vi "Acquisition Message Loop.vi"(8 "error in (no error)":errorcluster, 9 "Data Queue":refnum<queue>, 10 "Data Notifier":refnum<notifier>, 11 "Message Queues":T1) -> (0 "error out":errorcluster)   [LabVIEW 2017, in "Acquisition.lvlib"]
doc: "Message loop for handling messages pertaining to the acquisition of data from the hardware."
uses:
  Acquisition.lvlib
  support/Message Queue/All Message Queues.ctl
  support/Message Queue/Message Cluster.ctl
  Hardware Configuration.ctl
  <vilib>/DAQmx/read.llb/DAQmx Read (Analog 1D Wfm NChan NSamp).vi
  support/Message Queue/Enqueue Message (Single).vi
  <vilib>/DAQmx/miscellaneous.llb/DAQmx Fill In Error Info.vi
  <vilib>/Utility/error.llb/Error Cluster From Error Code.vi
  <vilib>/ErrorRing/Error Ring.xnode
  support/Message Queue/Message Queue.lvlib
  <resource>/objmgr/daqmx.rc
panel:
  out "# waiting":i32
  out "# elements in queue":i32
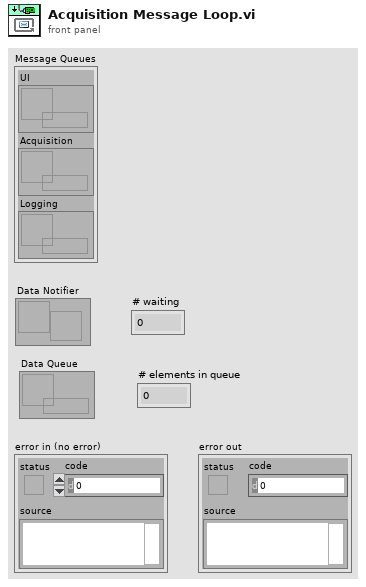
[diagram p1: front panel]
types:
  T1 = typedef "Message Queue.lvlib/All Message Queues.ctl" = cluster{"UI":refnum<queue>, "Acquisition":refnum<queue>, "Logging":refnum<queue>}
  T2 = typedef "Acquisition.lvlib/Hardware Configuration.ctl" = cluster{"DAQmx Input":tag, "Max Input":dbl, "Min Input":dbl, "Sample Rate":dbl, "DAQmx Task":refnum<k21>}
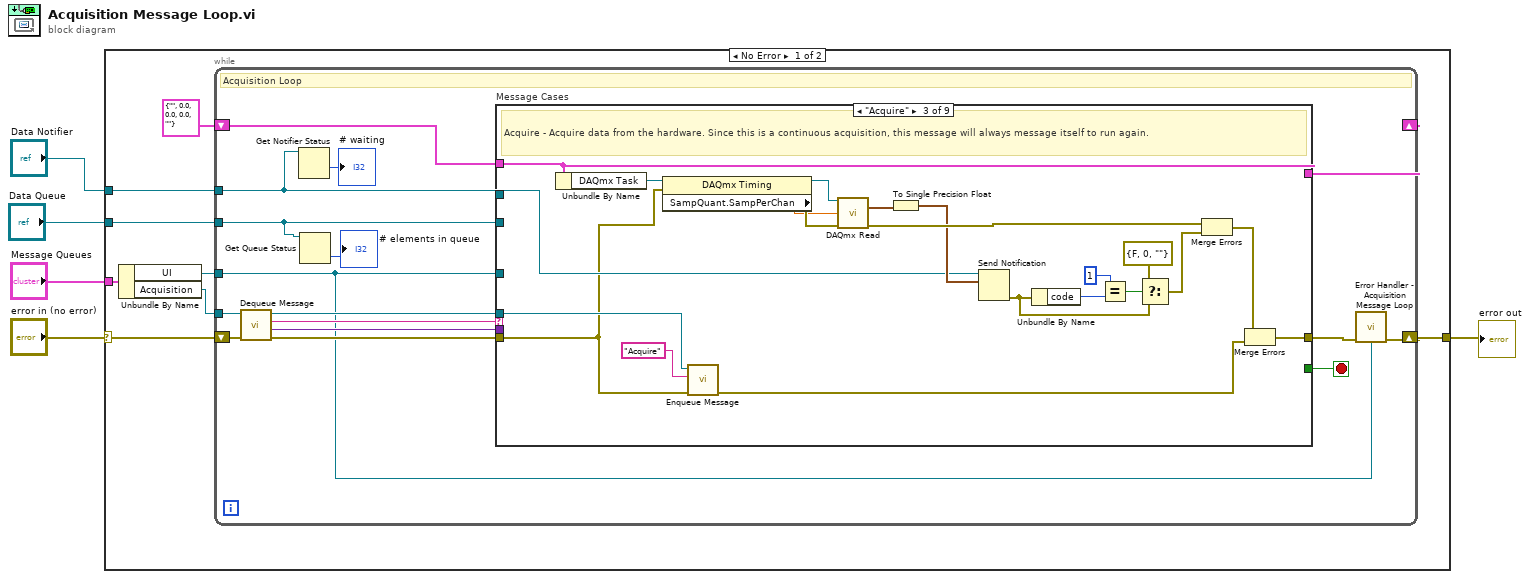
[diagram p0: block diagram]
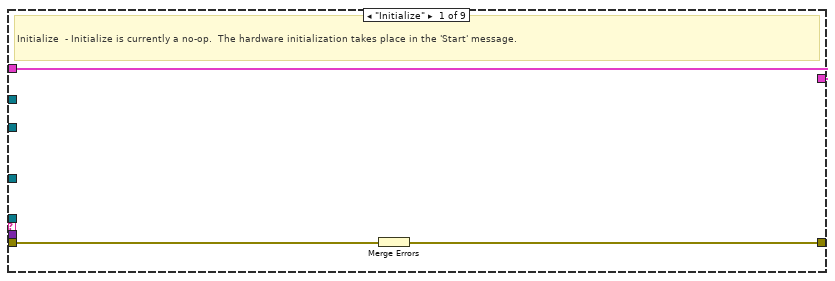
[diagram p2: hidden frame]
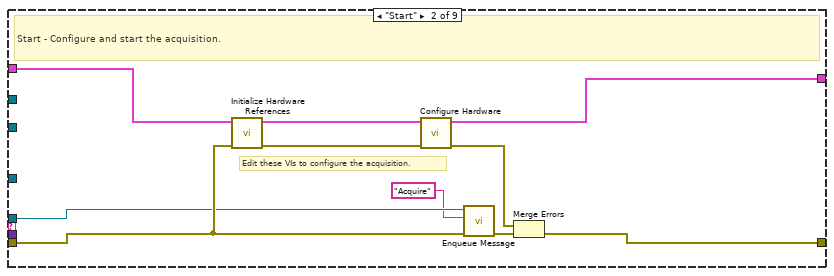
[diagram p3: hidden frame]
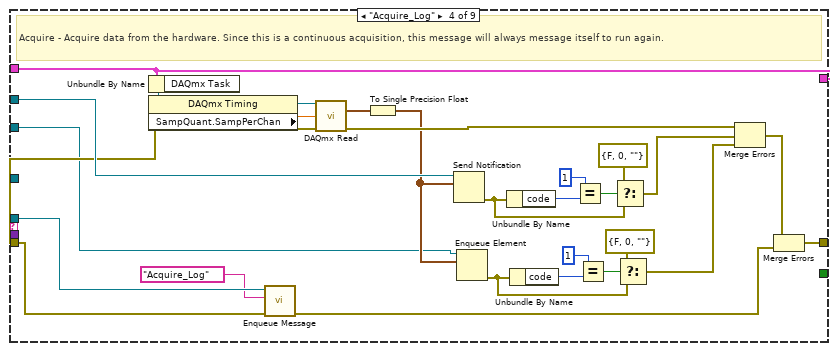
[diagram p4: hidden frame]
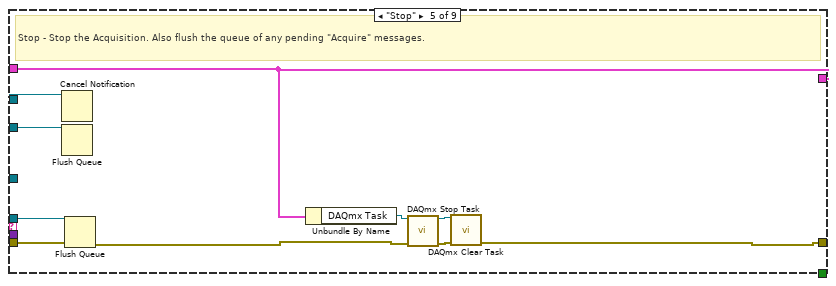
[diagram p5: hidden frame]
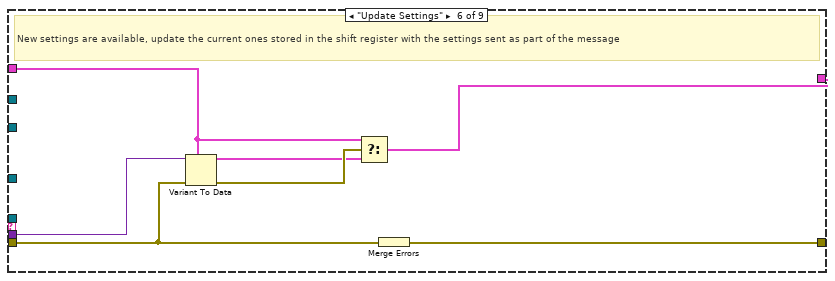
[diagram p6: hidden frame]
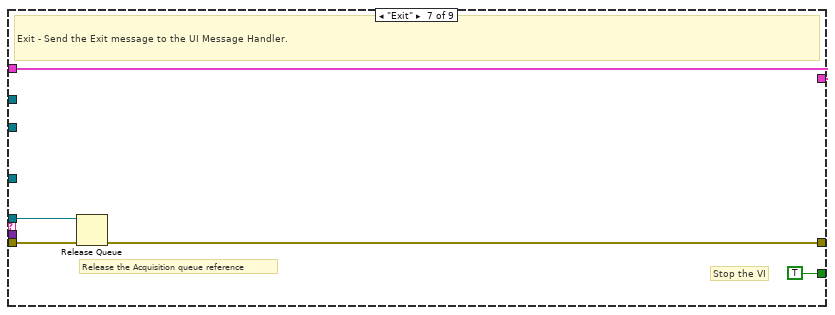
[diagram p7: hidden frame]
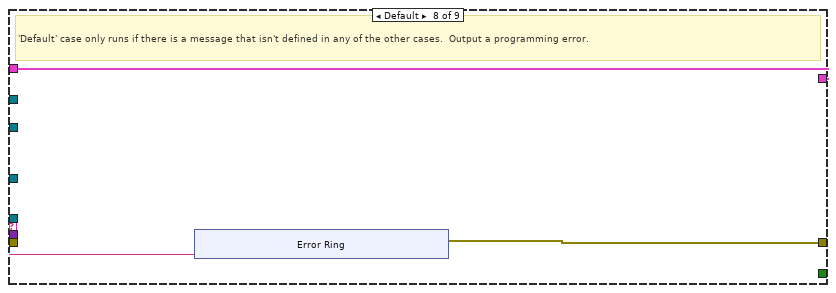
[diagram p8: hidden frame]
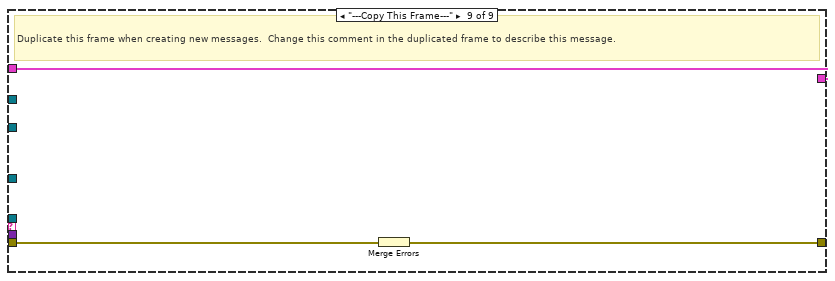
[diagram p9: hidden frame]
diagram:
  n1 = case shown="No Error" "error in (no error)" {
    selector: "error in (no error)" -> [w9 w127]
    tunnel: "Message Queues" -> [w13 _]
    tunnel: [w11 w127] -> w4
    tunnel: "Data Notifier" -> [w7 _]
    tunnel: "Data Queue" -> [w6 _]
    frame No Error {
      n2 = Unbundle By Name(w13) -> ("UI"=w8:refnum<queue>, "Acquisition"=w12:refnum<queue>)
      n3 = while {
        tunnel: w12 -> [w22]
        shift-right: [w18] -> _
        shift-left: T2 {"DAQmx Input"="", "Max Input"=0.0, "Min Input"=0.0, "Sample Rate"=0.0, "DAQmx Task"=""} ("Data Cluster") -> [w29]
        shift-right: [w20] -> w11
        shift-left: w9 -> [w27]
        tunnel: w8 -> [w19]
        tunnel: w7 -> [w16]
        tunnel: w6 -> [w14]
        stop <- w28 stop-if-true
        # "Acquisition Loop"
        n4 = call "Dequeue Message.vi"("error in (no error)"=w27, "Message Queue"=w22) -> ("error out"=w26:errorcluster, "Message Data"=w24:variant, "Message"=w25:string, "dup Message Queue"=w23:refnum<queue>)  [unwired: 6 in]
        n5 = Get Notifier Status(notifier=w16) -> (# waiting=→"# waiting":i32)  [unwired: 1 in, 4 out]
        n6 = Get Queue Status(queue=w14) -> (# elements in queue=→"# elements in queue":i32)  [unwired: 2 in, 7 out]
        n7 = case "Message Cases" shown="\"Acquire\"" w25 {
          selector: w25 -> [_ _ _ _ _ _ _ w116 _]
          tunnel: w23 -> [_ w39 w61 w89 w100 _ w111 _ _]
          tunnel: w26 -> [w31 w40 w44 w68 w101 w103 w112 _ w126]
          tunnel: [w32 w42 w63 w91 w92 w108 w109 w115 w125] -> w21
          tunnel: w29 -> [w30 w41 w43 w67 w94 w104 w110 w114 w124]
          tunnel: [_ _ _ _ _ _ TRUE _ _] -> w28
          tunnel: w24 -> [_ _ _ _ _ w107 _ _ _]
          tunnel: w19 -> [_ _ _ _ _ _ _ _ _]
          tunnel: w16 -> [_ _ w45 w69 w99 _ _ _ _]
          tunnel: [w30 w38 w43 w67 w94 w102 w110 w114 w124] -> w18
          tunnel: w14 -> [_ _ _ w64 w93 _ _ _ _]
          frame "Initialize" {
            # "Initialize  - Initialize is currently a no-op.  The hardware initialization takes place in the 'Start' message."
            n8 = Merge Errors(w31) -> (w32:errorcluster)
          }
          frame "Start" {
            # "Edit these VIs to configure the acquisition."
            # "Start - Configure and start the acquisition."
            n9 = call "Initialize Hardware References.vi"("error in (no error)"=w40, "Hardware Resources in"=w41) -> ("error out"=w33:errorcluster, "Hardware Resources out"=w34:T2)  [unwired: 8 in]
            n10 = call "Configure Hardware.vi"("error in (no error)"=w33, "Hardware Resources in"=w34) -> ("error out"=w36:errorcluster, "Hardware Resources out"=w38:T2)  [unwired: 8 in]
            n11 = call-poly "Enqueue Message.vi"("error in (no error)"=w40, "Message"="Acquire", "Message Queue"=w39) -> ("error out"=w37:errorcluster)  [unwired: 7 in, 1 out]
            n12 = Merge Errors(w36, w37) -> (w42:errorcluster)
          }
          frame "Acquire" {
            # "Acquire - Acquire data from the hardware. Since this is a continuous acquisition, this message will always message itself to run again."
            n13 = Unbundle By Name(w43) -> ("DAQmx Task"=w51:refnum<k21>)
            n14 = property class="DAQmx Timing"(reference=w51, error in=w44) -> (reference out=w50:refnum<k21>, error out=w49:errorcluster, "SampQuant.SampPerChan"=w48:dbl)
            n15 = call-poly "Enqueue Message.vi"("error in (no error)"=w44, "Message"="Acquire", "Message Queue"=w61) -> ("error out"=w62:errorcluster)  [unwired: 7 in, 1 out]
            n16 = call-poly <vilib>:"DAQmx Read.vi"("task/channels in"=w50, "number of samples per channel"=w48, "error in"=w49) -> ("data"=w52:waveform(dbl)[], "error out"=w53:errorcluster)  [unwired: 10 in, 1 out]
            n17 = To Single Precision Float(number=w52) -> (single precision float=w47:waveform(sgl)[])
            n18 = Send Notification(notification=w47, notifier=w45) -> (error out=w56:errorcluster)  [unwired: 1 in, 1 out]
            n19 = Unbundle By Name(w56) -> ("code"=w59:i32)
            n20 = Equal?(x=1, y=w59) -> (x = y?=w57:bool)
            n21 = Select(t=errorcluster {"status"=FALSE, "code"=0, "source"=""} ("error constant"), s=w57, f=w56) -> (s? t:f=w55:errorcluster)
            n22 = Merge Errors(w53, w55) -> (w46:errorcluster)
            n23 = Merge Errors(w46, w62) -> (w63:errorcluster)
          }
          frame "Acquire_Log" {
            # "Acquire - Acquire data from the hardware. Since this is a continuous acquisition, this message will always message itself to run again."
            n24 = Unbundle By Name(w67) -> ("DAQmx Task"=w74:refnum<k21>)
            n25 = property class="DAQmx Timing"(reference=w74, error in=w68) -> (reference out=w73:refnum<k21>, error out=w72:errorcluster, "SampQuant.SampPerChan"=w71:dbl)
            n26 = call-poly "Enqueue Message.vi"("error in (no error)"=w68, "Message"="Acquire_Log", "Message Queue"=w89) -> ("error out"=w90:errorcluster)  [unwired: 7 in, 1 out]
            n27 = call-poly <vilib>:"DAQmx Read.vi"("task/channels in"=w73, "number of samples per channel"=w71, "error in"=w72) -> ("data"=w66:waveform(dbl)[], "error out"=w75:errorcluster)  [unwired: 10 in, 1 out]
            n28 = To Single Precision Float(number=w66) -> (single precision float=w65:waveform(sgl)[])
            n29 = Send Notification(notification=w65, notifier=w69) -> (error out=w84:errorcluster)  [unwired: 1 in, 1 out]
            n30 = Enqueue Element(queue=w64, element=w65) -> (error out=w80:errorcluster)  [unwired: 2 in, 2 out]
            n31 = Unbundle By Name(w84) -> ("code"=w87:i32)
            n32 = Unbundle By Name(w80) -> ("code"=w77:i32)
            n33 = Equal?(x=1, y=w87) -> (x = y?=w85:bool)
            n34 = Equal?(x=1, y=w77) -> (x = y?=w79:bool)
            n35 = Select(t=errorcluster {"status"=FALSE, "code"=0, "source"=""} ("error constant"), s=w85, f=w84) -> (s? t:f=w83:errorcluster)
            n36 = Select(t=errorcluster {"status"=FALSE, "code"=0, "source"=""} ("error constant"), s=w79, f=w80) -> (s? t:f=w76:errorcluster)
            n37 = Merge Errors(w75, w83, w76) -> (w70:errorcluster)
            n38 = Merge Errors(w70, w90) -> (w91:errorcluster)
          }
          frame "Stop" {
            # "Stop - Stop the Acquisition. Also flush the queue of any pending \"Acquire\" messages."
            n39 = Cancel Notification(0:w99) -> ()  [unwired: 1 in, 3 out]
            n40 = Flush Queue(queue=w93) -> ()  [unwired: 1 in, 3 out]
            n41 = Flush Queue(queue=w100, error in (no error)=w101) -> (error out=w95:errorcluster)  [unwired: 2 out]
            n42 = Unbundle By Name(w94) -> ("DAQmx Task"=w98:refnum<k21>)
            n43 = call <vilib>:"DAQmx Stop Task.vi"("task/channels in"=w98, "error in"=w95) -> ("task out"=w97:refnum<k21>, "error out"=w96:errorcluster)  [unwired: 12 in]
            n44 = call <vilib>:"DAQmx Clear Task.vi"("task in"=w97, "error in"=w96) -> ("error out"=w92:errorcluster)  [unwired: 13 in]
          }
          frame "Update Settings" {
            # "New settings are available, update the current ones stored in the shift register with the settings sent as part of the message"
            n45 = Variant To Data(error in=w103, type=w104, Variant=w107) -> (data=w105:T2, error out=w106:errorcluster)
            n46 = Select(t=w104, s=w106, f=w105) -> (s? t:f=w102:T2)
            n47 = Merge Errors(w103) -> (w108:errorcluster)
          }
          frame "Exit" {
            # "Release the Acquisition queue reference"
            # "Stop the VI"
            # "Exit - Send the Exit message to the UI Message Handler."
            n48 = Release Queue(queue=w111, error in (no error)=w112) -> (error out=w109:errorcluster)  [unwired: 1 in, 2 out]
          }
          frame Default {
            # "'Default' case only runs if there is a message that isn't defined in any of the other cases.  Output a programming error."
            n49 = xnode "Error Ring"("parameter 0"=w116) -> ("error out"=w115:errorcluster)
          }
          frame "---Copy This Frame---" {
            # "Duplicate this frame when creating new messages.  Change this comment in the duplicated frame to describe this message."
            n50 = Merge Errors(w126) -> (w125:errorcluster)
          }
        }
        n51 = call "Error Handler - Acquisition Message Loop.vi"("error in (no error)"=w21, "Message Queue"=w19) -> ("dup error in"=w20:errorcluster)  [unwired: 8 in, 1 out]
      }
    }
    frame Error {
    }
  }
  "error out" <- w4
